vi "MGI Resettable Trigger (Reentrant).vi"(8 "error in (no error)":errorcluster, 9 "Reset (F)":bool, 10 "State":bool) -> (0 "error out":errorcluster, 1 "Triggered?":bool, 2 "Trigger":bool)   [LabVIEW 2020]
doc: "This VI sets the \"Trigger\" output high only once on a rising edge of the \"State\" input. The \"Triggered?\" output is high after the first time there is a rising edge on the \"State\" input. The trigger is resettable through the input \"Reset (F)\".\nThis VI is a reentrant functional global, so each instance of this VI refers to a different trigger.\n\nAuthored by David A. Moore\nsupport@mooregoodideas.com\nwww.mooregoodideas.com\n\nCopyright (c) 2010, Moore Good Ideas, Inc.\n\nAll rights reserved.\n\nRedistribution and use in source and binary forms, with or without modification, are permitted provided that the following conditions are met:\n\n * Redistributions of source code must retain the above copyright notice, this list of conditions and the following disclaimer.\n * Redistributions in binary form must reproduce the above copyright notice, this list of conditions and the following disclaimer in the documentation and/or other materials provided with the distribution.\n * Neither the name of Moore Good Ideas, Inc. nor the names of its contributors may be used to endorse or promote products derived from this software without specific prior written permission.\n\nTHIS SOFTWARE IS PROVIDED BY THE COPYRIGHT HOLDERS AND CONTRIBUTORS \"AS IS\" AND ANY EXPRESS OR IMPLIED WARRANTIES, INCLUDING, BUT NOT LIMITED TO, THE IMPLIED WARRANTIES OF MERCHANTABILITY AND FITNESS FOR A PARTICULAR PURPOSE ARE DISCLAIMED. IN NO EVENT SHALL THE COPYRIGHT OWNER OR CONTRIBUTORS BE LIABLE FOR ANY DIRECT, INDIRECT, INCIDENTAL, SPECIAL, EXEMPLARY, OR CONSEQUENTIAL DAMAGES (INCLUDING, BUT NOT LIMITED TO, PROCUREMENT OF SUBSTITUTE GOODS OR SERVICES; LOSS OF USE, DATA, OR PROFITS; OR BUSINESS INTERRUPTION) HOWEVER CAUSED AND ON ANY THEORY OF LIABILITY, WHETHER IN CONTRACT, STRICT LIABILITY, OR TORT (INCLUDING NEGLIGENCE OR OTHERWISE) ARISING IN ANY WAY OUT OF THE USE OF THIS SOFTWARE, EVEN IF ADVISED OF THE POSSIBILITY OF SUCH DAMAGE."
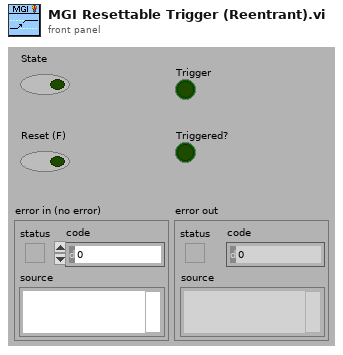
[diagram p1: front panel]
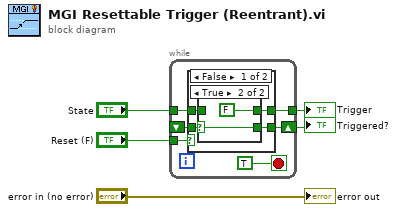
[diagram p0: block diagram]
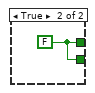
[diagram p3: hidden frame]
diagram:
  n1 = while {
    tunnel: "State" -> [w8]
    shift-right: [w10] -> w1
    shift-left: _ -> [w9]
    tunnel: [w7] -> w4
    tunnel: "Reset (F)" -> [w6]
    stop <- TRUE stop-if-true
    n2 = case shown="False" w6 {
      tunnel: [w14 w19] -> w10
      tunnel: w9 -> [w13 _]
      tunnel: w8 -> [w15 _]
      tunnel: [w12 w19] -> w7
      frame False {
        n3 = case shown="True" w13 {
          selector: w13 -> [_ w18]
          tunnel: w15 -> [w16 _]
          tunnel: [w16 w18] -> w14
          tunnel: [w16 FALSE ("State")] -> w12
          frame False {
          }
          frame True {
          }
        }
      }
      frame True {
        w19 = FALSE ("State")
      }
    }
  }
  "Trigger" <- w4
  "Triggered?" <- w1
  "error out" <- "error in (no error)"
